vi "Agilent set frequency.vi"(7 "Frequency GHz":dbl, 8 "error in (no error)":errorcluster, 11 "VISA resource name":refnum<visa-resource-name>) -> (0 "error out":errorcluster, 3 "VISA resource name out":refnum<visa-resource-name>)   [LabVIEW 2024]
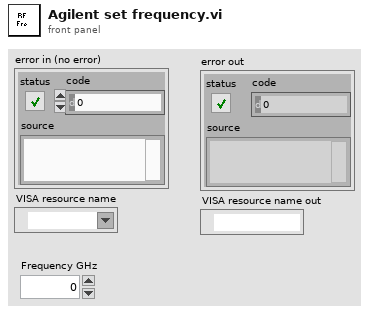
[diagram p1: front panel]
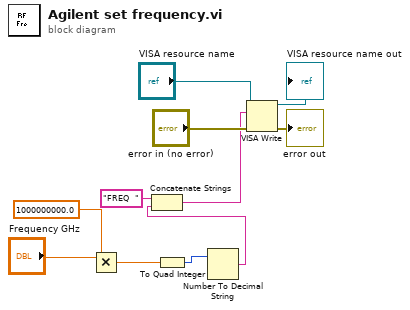
[diagram p0: block diagram]
diagram:
  n1 = Multiply(x="Frequency GHz", y=1000000000.0) -> (x*y=w3:dbl)
  n2 = To Quad Integer(1:w3) -> (0:w2:i64)
  n3 = Number To Decimal String(number=w2) -> (decimal integer string=w1:string)  [unwired: 1 in]
  n4 = Concatenate Strings("FREQ  " ("string"), w1) -> (w6:string)
  n5 = VISA Write(VISA resource name="VISA resource name", write buffer=w6, error in (no error)="error in (no error)") -> (VISA resource name out=→"VISA resource name out":refnum<visa-resource-name>, error out=→"error out":errorcluster)  [unwired: 1 out]
